vi "BallShear_main.vi"() -> ()   [LabVIEW 2013]
uses:
  System.Windows.Forms
panel:
  out "Numeric":i32
  in  "Options":enum32{"Shear", "Settings"}(tab)
  out "Ball Selected":dbl
  in  "Shear Speed":dbl
  out "Total Steps":dbl
  in  "Check":bool
  out "Ready":bool
  in  "Remove Package":bool
  in  "Proceed":bool
  in  "Preceed":bool
  out "PictureBox":refnum<k24>(container)
  out "Step":dbl
  in  "Image Path":path
  in  "Image Name":string
  in  "Displayed Image":path
  out "Ready":bool
  in  "Power":bool=TRUE
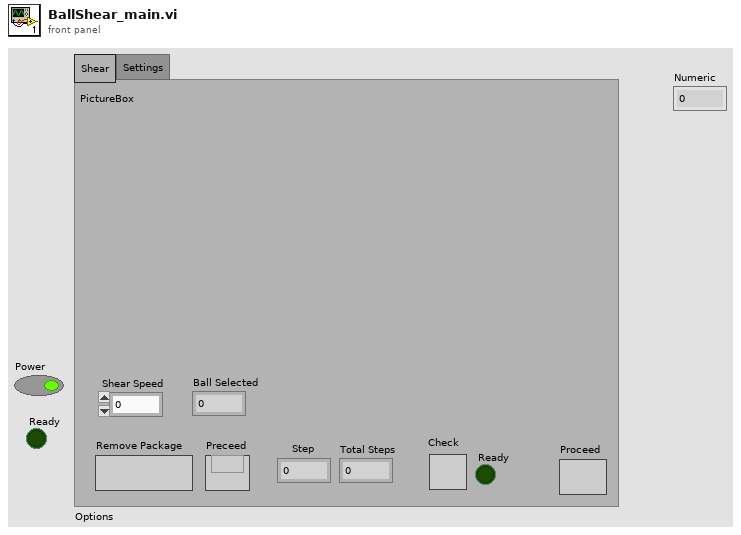
[diagram p1: front panel]
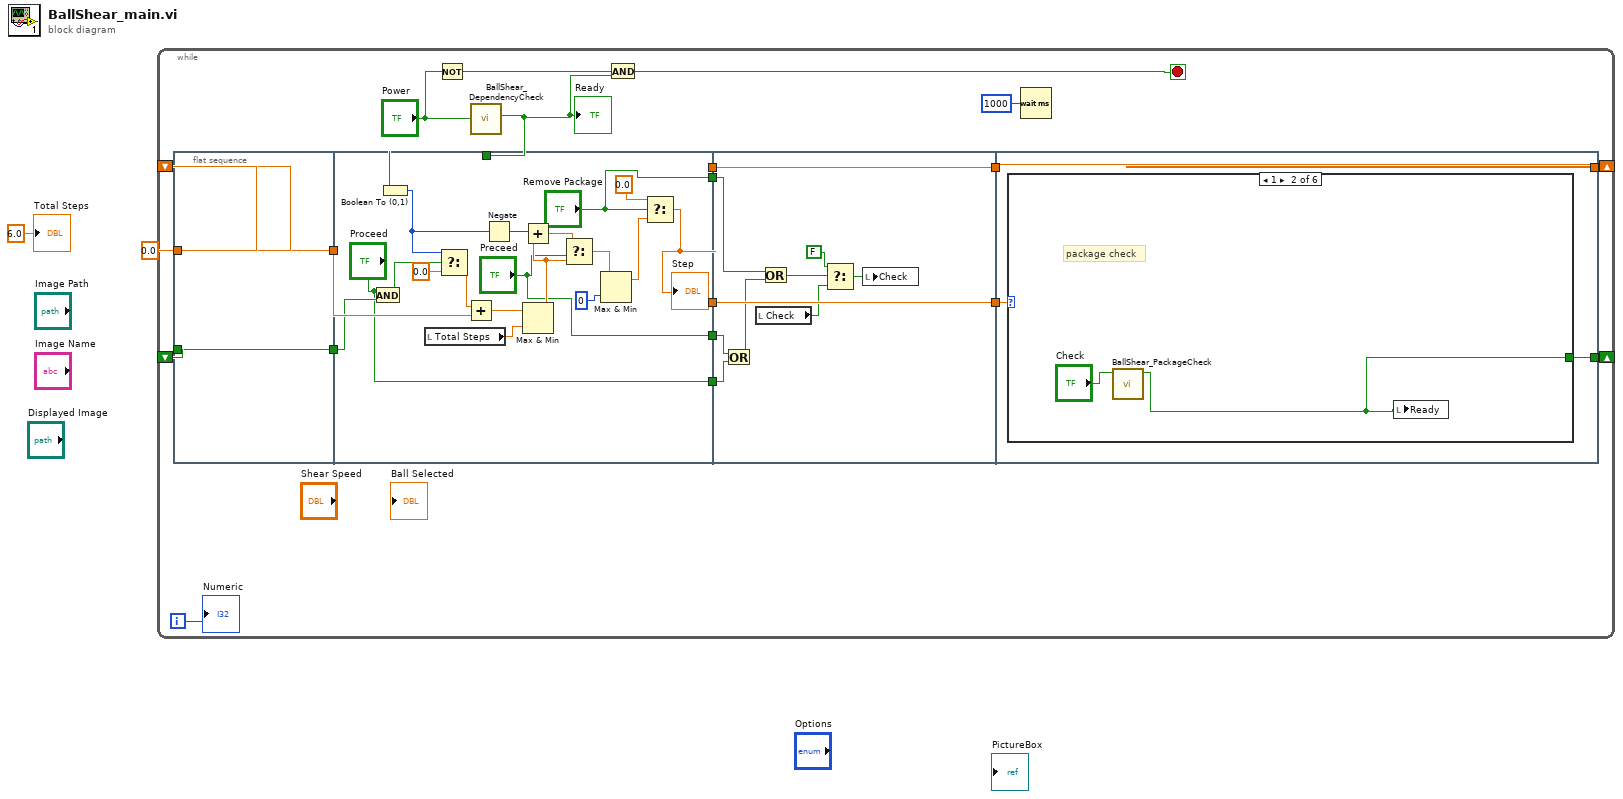
[diagram p0: block diagram]
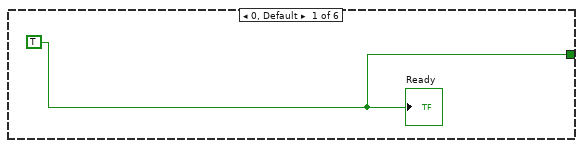
[diagram p2: hidden frame]
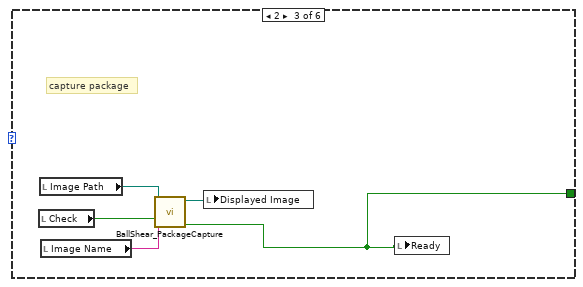
[diagram p3: hidden frame]
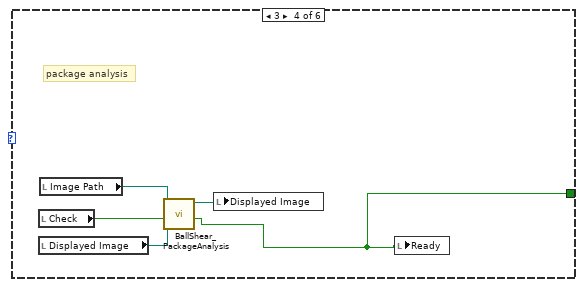
[diagram p4: hidden frame]
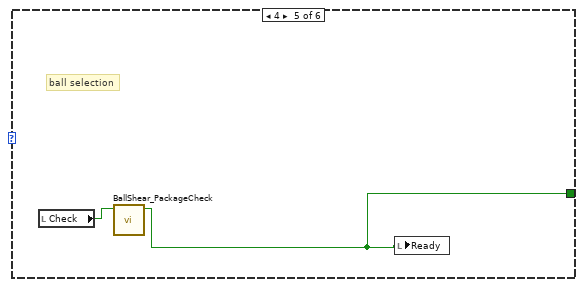
[diagram p5: hidden frame]
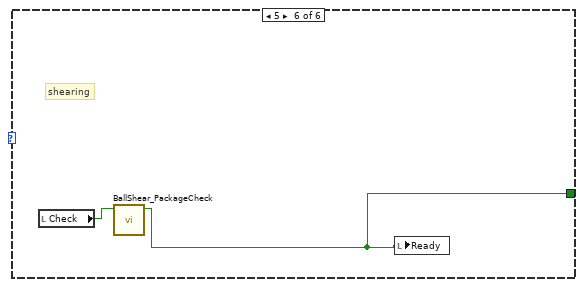
[diagram p6: hidden frame]
diagram:
  n1 = while {
    shift-right: [w14] -> _
    shift-left: 0.0 ("Step") -> [w16]
    shift-right: [w12] -> _
    shift-left: _ -> [w10]
    i -> [w17]
    stop <- w19 stop-if-true
    n2 = flat-sequence {
      tunnel: w16 -> [w23]
      tunnel: [w23] -> w13
      tunnel: [w22] -> w11
      tunnel: w10 -> [w22]
      tunnel: w15 -> [w38]
      tunnel: [w29] -> w9
      tunnel: w13 -> [w39]
      tunnel: [w29] -> w7
      tunnel: w11 -> [w28]
      tunnel: ["Remove Package"] -> w5
      tunnel: ["Proceed"] -> w4
      tunnel: ["Preceed"] -> w3
      tunnel: w9 -> [w53]
      tunnel: [w53] -> w8
      tunnel: w7 -> [w52]
      tunnel: [w52] -> w6
      tunnel: w5 -> [w49]
      tunnel: w4 -> [w50]
      tunnel: w3 -> [w51]
      tunnel: [w56] -> w14
      tunnel: w8 -> [w56]
      tunnel: w6 -> [w55]
      tunnel: [w54] -> w12
      frame #0 {
      }
      frame #1 {
        n3 = And(x="Proceed", y=w28) -> (x .and. y?=w27:bool)
        n4 = Boolean To (0,1)(Boolean=w38) -> (0, 1=w37:i16)
        n5 = local read "Total Steps"() -> (w31:dbl)
        n6 = Select(t=w37, s=w27, f=0.0) -> (s? t:f=w41:dbl)
        n7 = Add(x=w41, y=w39) -> (x+y=w36:dbl)
        n8 = Negate(x=w37) -> (-x=w42:i16)
        n9 = Max & Min(x=w36, y=w31) -> (min(x,y)=w35:dbl)  [unwired: 1 out]
        n10 = Add(x=w42, y=w35) -> (x+y=w43:dbl)
        n11 = Select(t=w43, s="Preceed", f=w35) -> (s? t:f=w34:dbl)
        n12 = Max & Min(x=w34, y=i16 0) -> (max(x,y)=w33:dbl)  [unwired: 1 out]
        n13 = Select(t=0.0, s="Remove Package", f=w33) -> (s? t:f=w29:dbl)
        "Step" <- w29
      }
      frame #2 {
        n14 = Or(x=w51, y=w50) -> (x .or. y?=w48:bool)
        n15 = local read "Check"() -> (w45:bool)
        n16 = Or(x=w49, y=w48) -> (x .or. y?=w47:bool)
        n17 = Select(t=FALSE, s=w47, f=w45) -> (s? t:f=w44:bool)
        n18 = local write "Check"(w44) -> ()
      }
      frame #3 {
        n19 = case shown="1" w55 {
          tunnel: [w57 w58 w64 w67 w71 w73] -> w54
          frame 0, Default {
            w57 = TRUE
            "Ready" <- w57
          }
          frame 1 {
            # "package check"
            n20 = call "BallShear_PackageCheck.vi"("Check"="Check") -> ("Ready"=w58:bool)  [unwired: 10 in]
            n21 = local write "Ready"(w58) -> ()
          }
          frame 2 {
            # "capture package"
            n22 = local read "Check"() -> (w61:bool)
            n23 = local read "Image Path"() -> (w63:path)
            n24 = local read "Image Name"() -> (w62:string)
            n25 = call "BallShear_PackageCapture.vi"("Target Name"=w62, "Capture"=w61, "Target Path"=w63) -> ("Success"=w64:bool, "Actual Image Path"=w60:path)  [unwired: 7 in]
            n26 = local write "Displayed Image"(w60) -> ()
            n27 = local write "Ready"(w64) -> ()
          }
          frame 3 {
            # "package analysis"
            n28 = local read "Check"() -> (w68:bool)
            n29 = local read "Displayed Image"() -> (w65:path)
            n30 = local read "Image Path"() -> (w69:path)
            n31 = call "BallShear_PackageAnalysis.vi"("Original Image Path"=w65, "Analyze"=w68, "Image Directory"=w69) -> ("Success"=w67:bool, "Analyzed Image Path"=w66:path)  [unwired: 7 in]
            n32 = local write "Displayed Image"(w66) -> ()
            n33 = local write "Ready"(w67) -> ()
          }
          frame 4 {
            # "ball selection"
            n34 = local read "Check"() -> (w70:bool)
            n35 = call "BallShear_PackageCheck.vi"("Check"=w70) -> ("Ready"=w71:bool)  [unwired: 10 in]
            n36 = local write "Ready"(w71) -> ()
          }
          frame 5 {
            # "shearing"
            n37 = local read "Check"() -> (w72:bool)
            n38 = call "BallShear_PackageCheck.vi"("Check"=w72) -> ("Ready"=w73:bool)  [unwired: 10 in]
            n39 = local write "Ready"(w73) -> ()
          }
        }
      }
    }
    n40 = Not(x="Power") -> (.not. x?=w20:bool)
    n41 = call "BallShear_DependencyCheck.vi"("Power"="Power") -> ("Ready"=w15:bool)  [unwired: 10 in]
    "Ready" <- w15
    n42 = And(x=w20, y=w15) -> (x .and. y?=w19:bool)
    n43 = Wait (ms)(milliseconds to wait=u32 1000) -> ()  [unwired: 1 out]
    "Numeric" <- w17
  }
  "Total Steps" <- 6.0 ("Total Steps")
